vi "Doubles Events (SubVI).vi"(1 "Singles Events":string, 2 "PLAYER NAMES":string[](array[string])) -> (0 "Edited Events For Doubles":string)   [LabVIEW 2013]
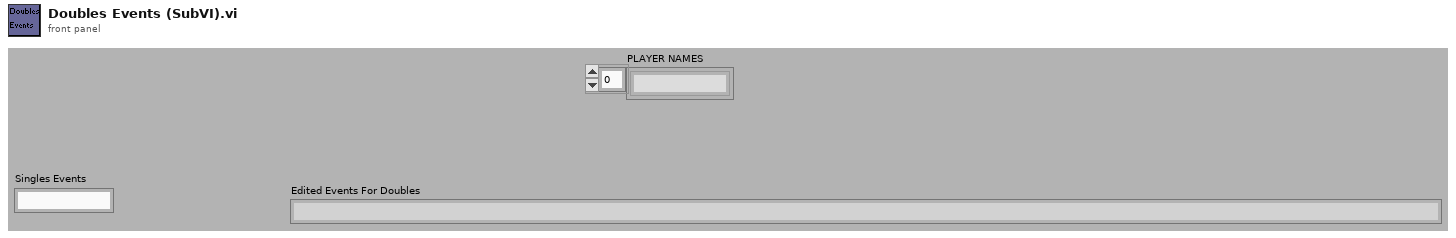
[diagram p1: front panel]
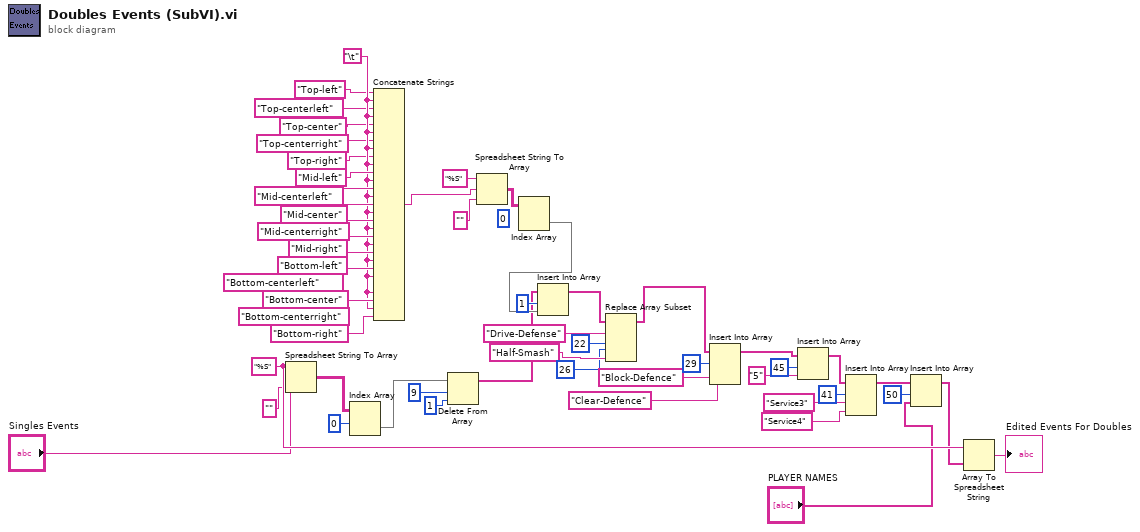
[diagram p0: block diagram]
diagram:
  (unwired) 0 ("index (row)")
  w18 = "\t"
  w51 = "%S" ("format string")
  n1 = Spreadsheet String To Array(format string=w51, spreadsheet string="Singles Events", array type (2D Dbl)="") -> (array=w12:string[][])  [unwired: 1 in]
  n2 = Index Array(array=w12, index (row)=0) -> (element=w32:string[])  [unwired: 1 in]
  n3 = Concatenate Strings("Top-left" ("string"), w18, "Top-centerleft" ("string"), w18, "Top-center" ("string"), w18, "Top-centerright" ("string"), w18, "Top-right" ("string"), w18, "Mid-left" ("string"), w18, "Mid-centerleft" ("string"), w18, "Mid-center" ("string"), w18, "Mid-centerright" ("string"), w18, "Mid-right" ("string"), w18, "Bottom-left" ("string"), w18, "Bottom-centerleft" ("string"), w18, "Bottom-center" ("string"), w18, "Bottom-centerright" ("string"), w18, "Bottom-right" ("string")) -> (w31:string)
  n4 = Delete From Array(array=w32, length=9, index=1 ("index 2")) -> (array with subset deleted=w35:string[])  [unwired: 1 out]
  n5 = Spreadsheet String To Array(format string="%S", spreadsheet string=w31, array type (2D Dbl)="") -> (array=w36:string[][])  [unwired: 1 in]
  n6 = Index Array(array=w36) -> (element=w37:string[])  [unwired: 2 in]
  n7 = Insert Into Array(array=w35, index=1, new element=w37) -> (w39:string[])
  n8 = Replace Array Subset(array=w39, new element #1="Drive-Defense" ("new element/subarray"), index #1=22 ("index"), new element #2="Half-Smash" ("new element/subarray"), index #2=26 ("index")) -> (w43:string[])
  n9 = Insert Into Array(array=w43, index=29, new element #1="Block-Defence" ("new element/subarray"), new element #2="Clear-Defence" ("new element/subarray")) -> (w47:string[])
  n10 = Insert Into Array(array=w47, index=45, new element="5" ("new element/subarray")) -> (w5:string[])
  n11 = Insert Into Array(array=w5, index=41, new element #1="Service3" ("new element/subarray"), new element #2="Service4" ("new element/subarray")) -> (w3:string[])
  n12 = Insert Into Array(array=w3, index=50, new element="PLAYER NAMES") -> (w1:string[])
  n13 = Array To Spreadsheet String(array=w1, 3:w51) -> (spreadsheet string=→"Edited Events For Doubles":string)  [unwired: 1 in]
